vi "Change File Extension (SubVI).vi"(10 "New Extension":string="temp", 11 "appended path":path) -> (1 "New file path":path, 2 "stripped path":path, 3 "Original Path":path)   [LabVIEW 2019]
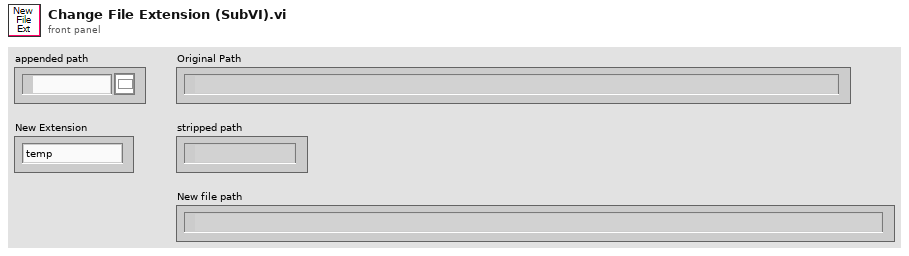
[diagram p1: front panel]
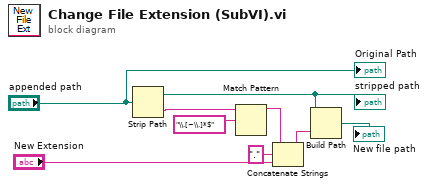
[diagram p0: block diagram]
diagram:
  n1 = Strip Path(path="appended path") -> (stripped path=w4:path, name=w3:string)
  "stripped path" <- w4
  n2 = Match Pattern(string=w3, regular expression="\\.[~\\.]*$") -> (before substring=w5:string)  [unwired: 4 out]
  n3 = Concatenate Strings(w5, "." ("string"), "New Extension") -> (w8:string)
  n4 = Build Path(base path=w4, name or relative path=w8) -> (appended path=→"New file path":path)
  "Original Path" <- "appended path"
